vi "Arms SSS.vi"(11 "Arms SS Actuator Values 2":T1) -> (3 "Arms SS Actuator Values":T1)   [LabVIEW 2014]
uses:
  Arms SS Typedef.ctl
  <vilib>/Rock Robotics/WPI/Solenoid/WPI_SolenoidValue.ctl
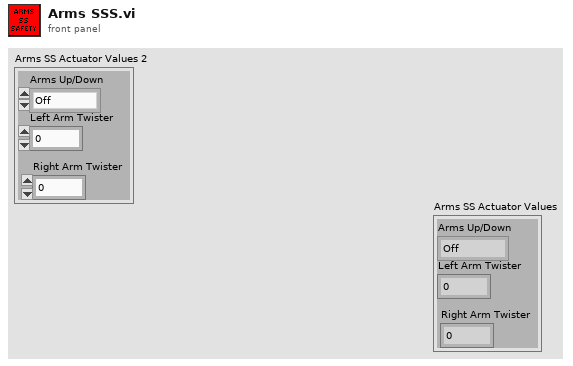
[diagram p1: front panel]
types:
  T1 = typedef "Arms SS Typedef.ctl" = cluster{"Arms Up/Down":T2, "Left Arm Twister":dbl, "Right Arm Twister":dbl}
  T2 = typedef "WPI_SolenoidValue.ctl" = enum16{"Off", "On", "Forward", "Reverse"}
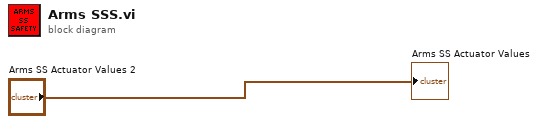
[diagram p0: block diagram]
diagram:
  "Arms SS Actuator Values" <- "Arms SS Actuator Values 2"
